vi "Servicio seleccionado.vi"(8 "error in (no error)":errorcluster, 10 "Servicio":string, 11 "Paquetes in":refnum<class "Paquetes.lvclass">) -> (0 "error out":errorcluster, 3 "Paquetes out":refnum<class "Paquetes.lvclass">)   [LabVIEW 2020, in "Paquetes.lvlib" / "Paquetes.lvclass"]
uses:
  Paquetes.lvclass
  C:/Program Files (x86)/National Instruments/LabVIEW 2020/vi.lib/ActorFramework/Actor/Actor.lvclass
  <vilib>/ActorFramework/Actor/Actor.lvclass/Actor.ctl
  Paquetes.lvclass/Paquetes.ctl
  UI Messages/Obtain servicio from paquetes Msg/Obtain servicio from paquetes Msg.lvclass/Obtain servicio from paquetes Msg.ctl
  <vilib>/ActorFramework/Message Enqueuer/Message Enqueuer.lvclass/Message Enqueuer.ctl
  <vilib>/ActorFramework/Message Enqueuer/Enqueue.vi
  UI Messages/Obtain servicio from paquetes Msg/Obtain servicio from paquetes Msg.lvclass
  C:/Program Files (x86)/National Instruments/LabVIEW 2020/vi.lib/ActorFramework/Message/Message.lvclass
  <vilib>/ActorFramework/Message Priority Queue/Priority Enqueue.vi
  <vilib>/ActorFramework/Actor/Actor.lvclass
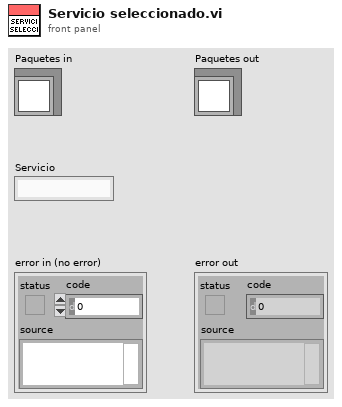
[diagram p1: front panel]
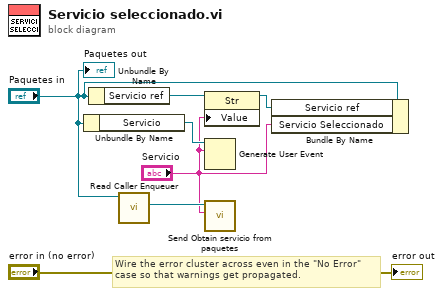
[diagram p0: block diagram]
diagram:
  # "Wire the error cluster across even in the \"No Error\"\ncase so that warnings get propagated."
  n1 = Unbundle By Name("Paquetes in") -> ("Servicio"=w4:refnum<user-event>)
  n2 = Unbundle By Name("Paquetes in") -> ("Servicio ref"=w6:refnum<vi>)
  n3 = call <vilib>:"Read Caller Enqueuer.vi"("Actor"="Paquetes in") -> ("Caller Enqueuer"=w2:refnum<class "Message Enqueuer.lvclass">)  [unwired: 10 in]
  n4 = property class="Str"(reference=w6, "Value"="Servicio") -> (reference out=w5:refnum<vi>)  [unwired: 1 in, 1 out]
  n5 = Generate User Event(user event=w4, event data cluster="Servicio") -> ()  [unwired: 2 in, 2 out]
  n6 = call "Send Obtain servicio from paquetes.vi"("Servicio seleccionado"="Servicio", "Message Enqueuer"=w2) -> ()  [unwired: 8 in, 2 out]
  n7 = Bundle By Name(cluster="Paquetes in", "Servicio ref"=w5, "Servicio Seleccionado"="Servicio") -> ()  [unwired: 1 out]
  "error out" <- "error in (no error)"
  "Paquetes out" <- "Paquetes in"
